vi "Set Channel PWM.vi"(8 "error in (no error)":errorcluster, 9 "Channel":u8, 10 "Duty Cycle 50%)":dbl=50.0, 11 "PWM in":refnum<class "LINX-PCA9685 PWM.lvclass">) -> (0 "error out":errorcluster, 3 "PWM out":refnum<class "LINX-PCA9685 PWM.lvclass">)   [LabVIEW 2020, in "LINX-PCA9685 PWM.lvclass"]
doc: "Sets the duty cycle (0-100%) of the specified channel (0-15)."
uses:
  LINX-PCA9685 PWM.lvclass
  LINX I2C/LINX I2C.lvclass
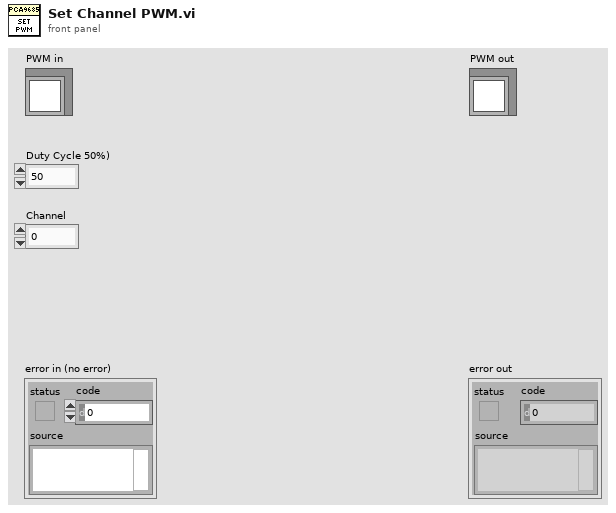
[diagram p1: front panel]
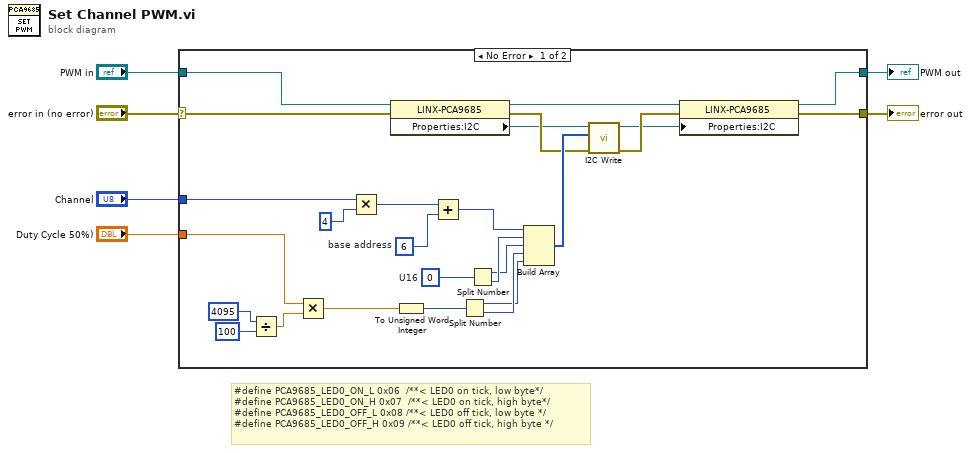
[diagram p0: block diagram]
diagram:
  # "#define PCA9685_LED0_ON_L 0x06  /**< LED0 on tick, low byte*/\n#define PCA9685_LED0_ON_H 0x07  /**< LED0 on tick, high byte*/\n#define PCA9685_LED0_OFF_L 0x08 /**< LED0 off tick, low byte */\n#define PCA9685_LED0_OFF_H 0x09 /**< LED0 off tick, high byte */"
  n1 = case shown="No Error" "error in (no error)" {
    selector: "error in (no error)" -> [w11 w33]
    tunnel: [w31 w33] -> w5
    tunnel: [w8 w32] -> w3
    tunnel: "PWM in" -> [w12 w32]
    tunnel: "Channel" -> [w30 _]
    tunnel: "Duty Cycle 50%)" -> [w21 _]
    frame No Error {
      w20 = u16 0  # U16
      w27 = u8 6  # base address
      n2 = Divide(x=4095, y=100) -> (x/y=w22:dbl)
      n3 = Multiply(x=w21, y=w22) -> (x*y=w17:dbl)
      n4 = Multiply(x=w30, y=u8 4) -> (x*y=w28:u8)
      n5 = property class="LINX-PCA9685"(reference=w12, error in=w11) -> (reference out=w13:refnum<class "LINX-PCA9685 PWM.lvclass">, error out=w10:errorcluster, "Properties:I2C"=w9:refnum<class "LINX I2C.lvclass">)
      n6 = To Unsigned Word Integer(number=w17) -> (unsigned 16bit integer=w16:u16)
      n7 = Add(x=w28, y=w27) -> (x+y=w26:u8)
      n8 = Split Number(x=w16) -> (hi(x)=w14:u8, lo(x)=w15:u8)
      n9 = Split Number(x=w20) -> (hi(x)=w18:u8, lo(x)=w19:u8)
      n10 = Build Array(w26, w19, w18, w15, w14) -> (w25:u8[])
      n11 = call "I2C Write.vi"("error in (no error)"=w10, "Bytes to Write"=w25, "LINX I2C in"=w9) -> ("error out"=w31:errorcluster, "LINX I2C out"=w7:refnum<class "LINX I2C.lvclass">)  [unwired: 7 in]
      n12 = property class="LINX-PCA9685"(reference=w13, "Properties:I2C"=w7) -> (reference out=w8:refnum<class "LINX-PCA9685 PWM.lvclass">)  [unwired: 1 in, 1 out]
    }
    frame Error {
    }
  }
  "error out" <- w5
  "PWM out" <- w3
